vi "Rotating and using Text.vi"() -> ()   [LabVIEW 2023]
doc: "This VI demonstrates how to display text in a 3D Picture with the Create Text with Alignment VI."
uses:
  <vilib>/Utility/miscctls.llb/LVSceneTextAlignment.ctl
  <vilib>/picture/3D Picture Control/Object/Create Object (drawable).vi
  <vilib>/picture/3D Picture Control/Helpers/Apply Texture (no reference).vi
  <vilib>/picture/3D Picture Control/Object/Add Object (no reference).vi
  <vilib>/picture/3D Picture Control/Object/Add Object (reference).vi
  <vilib>/picture/3D Picture Control/NI_3D Picture Control.lvlib
panel:
  in  "Text":string="LabVIEW"
  in  "Stop":bool
  out "3D Picture":refnum<vi>(3d-picture)
  # "Overview: This VI demonstrates how to display text in a 3D Picture with the Create Text with Alignment VI. \nRequirements: LabVIEW Full Development System\nInstructions:\n1. Run the VI. You will see the Text value as a texture on the cube and as several separate objects around the cube.\n2. Click Stop to stop the VI."
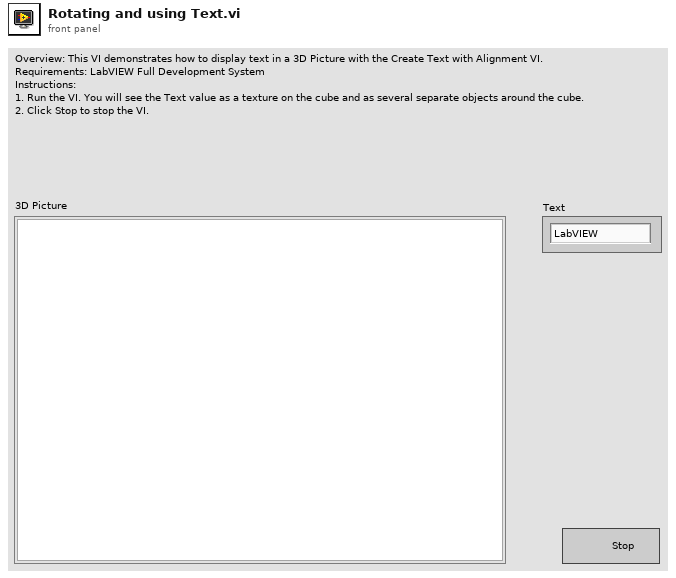
[diagram p1: front panel]
types:
  T1 = typedef "LVSceneTextAlignment.ctl" = cluster{"Horizontal Alignment":enum8{"Left", "Right", "Center"}, "Vertical Alignment":enum8{"Top", "Bottom", "Center", "Base Line", "Bottom Base Line"}}
  T2 = cluster{"Alignment":T1, "Axis Alignment":enum8{"X-Y", "Y-Z", "X-Z", "Reversed X-Y", "Reversed Y-Z", "Reversed X-Z", "Screen"}, "Vertical?":bool, "Wrap Distance":sgl}
  T3 = cluster{"horizontal":enum16{"left", "center", "right"}, "vertical":enum16{"top", "center", "bottom"}}
  T4 = enum16{"As a Decal", "With Modulation", "With Blending", "As a replacement"}
  T5 = cluster{"left":i16, "top":i16, "right":i16, "bottom":i16}
  T6 = typedef "imagedata.ctl" = cluster{"image type":i32, "image depth":i32, "image":u8[], "mask":u8[], "colors":u32[], "Rectangle":cluster{"left":i16, "top":i16, "right":i16, "bottom":i16}}
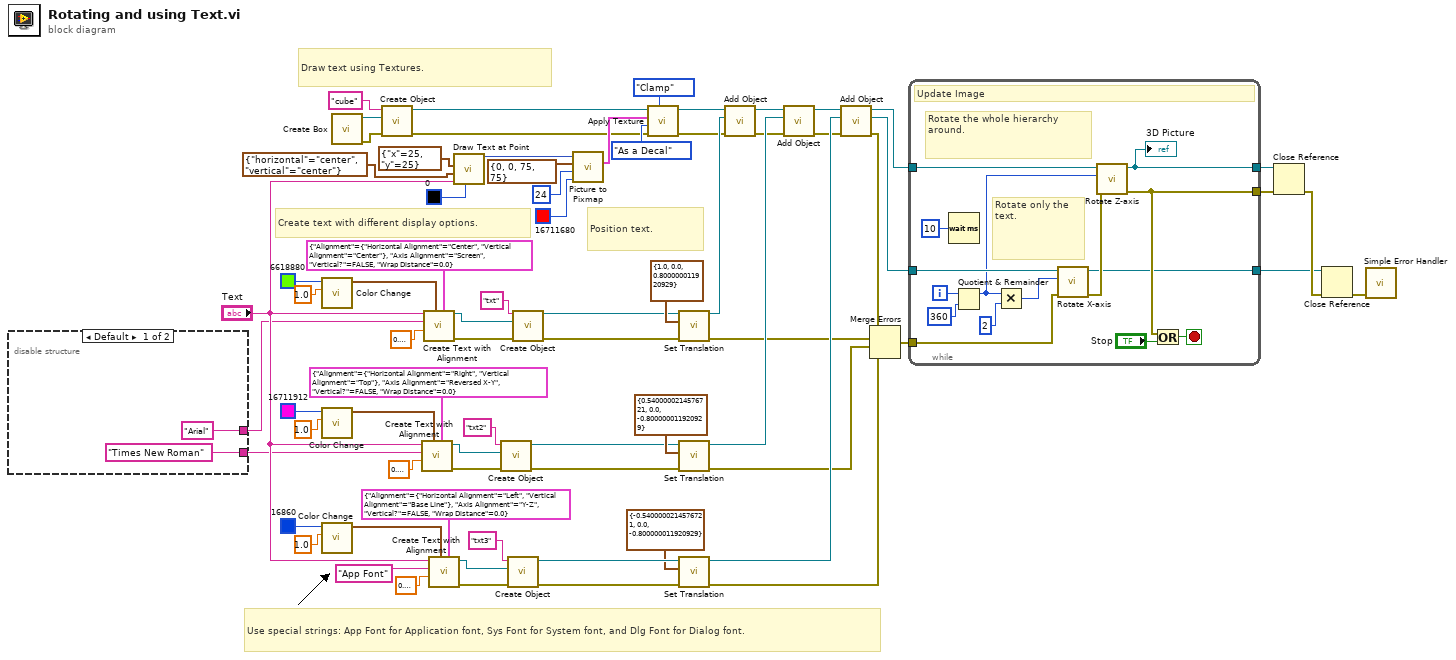
[diagram p0: block diagram]
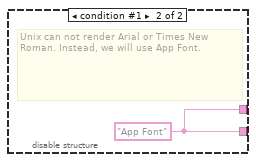
[diagram p2: hidden frame]
diagram:
  # "Use special strings: App Font for Application font, Sys Font for System font, and Dlg Font for Dialog font."
  # "Create text with different display options."
  # "Position text."
  # "Draw text using Textures."
  n1 = disable-structure shown="Default" {
    disable-tunnel: ["Arial" ("pattern") w76] -> w2
    disable-tunnel: ["Times New Roman" ("pattern") w76] -> w1
    frame condition #0 (active) {
    }
    frame condition #1 {
      w76 = "App Font" ("pattern")
      # "Unix can not render Arial or Times New Roman. Instead, we will use App Font."
    }
  }
  n2 = call <vilib>:"Color Change.vi"("Alpha"=1.0, "Color"=u32 6618880) -> ("RGBA"=w70:cluster{"R":sgl, "G":sgl, "B":sgl, "A":sgl})  [unwired: 9 in]
  n3 = call <vilib>:"Color Change.vi"("Alpha"=1.0, "Color"=u32 16711912) -> ("RGBA"=w46:cluster{"R":sgl, "G":sgl, "B":sgl, "A":sgl})  [unwired: 9 in]
  n4 = call <vilib>:"Color Change.vi"("Alpha"=1.0, "Color"=u32 16860) -> ("RGBA"=w33:cluster{"R":sgl, "G":sgl, "B":sgl, "A":sgl})  [unwired: 9 in]
  n5 = call <vilib>:"Create Box.vi"() -> ("error out"=w24:errorcluster, "New Box Refnum"=w73:refnum<vi>)  [unwired: 10 in]
  n6 = call-poly <vilib>:"Create Object.vi"("error in (no error)"=w24, "Geometry"=w73, "Name"="cube") -> ("error out"=w23:errorcluster, "Scene:New Object"=w57:refnum<vi>)  [unwired: 7 in]
  n7 = call <vilib>:"Create Text with Alignment.vi"("Font Options"=T2 {"Alignment"={"Horizontal Alignment"=enum."Right", "Vertical Alignment"=enum."Top"}, "Axis Alignment"=enum."Reversed X-Y", "Vertical?"=FALSE, "Wrap Distance"=0.0} ("Font options"), "Color"=w46, "Character Size"=sgl 0.3, "Font Name"=w1, "Text"="Text") -> ("error out"=w16:errorcluster, "New Text Refnum"=w42:refnum<vi>)  [unwired: 5 in]
  n8 = call <vilib>:"Create Text with Alignment.vi"("Font Options"=T2 {"Alignment"={"Horizontal Alignment"=enum."Center", "Vertical Alignment"=enum."Center"}, "Axis Alignment"=enum."Screen", "Vertical?"=FALSE, "Wrap Distance"=0.0} ("Font options"), "Color"=w70, "Character Size"=sgl 0.2, "Font Name"=w2, "Text"="Text") -> ("error out"=w18:errorcluster, "New Text Refnum"=w55:refnum<vi>)  [unwired: 5 in]
  n9 = call <vilib>:"Create Text with Alignment.vi"("Font Options"=T2 {"Alignment"={"Horizontal Alignment"=enum."Left", "Vertical Alignment"=enum."Base Line"}, "Axis Alignment"=enum."Y-Z", "Vertical?"=FALSE, "Wrap Distance"=0.0} ("Font options"), "Color"=w33, "Character Size"=sgl 0.2, "Font Name"="App Font" ("pattern"), "Text"="Text") -> ("error out"=w14:errorcluster, "New Text Refnum"=w36:refnum<vi>)  [unwired: 5 in]
  n10 = call <vilib>:"Draw Text at Point.vi"("text color(black)"=u32 0, "text"="Text", "alignment(left, top)"=T3 {"horizontal"=enum."center", "vertical"=enum."center"}, "origin"=cluster{"x":i16, "y":i16} {"x"=25, "y"=25}) -> ("new picture"=w63:picture)  [unwired: 6 in, 1 out]
  n11 = call-poly <vilib>:"Create Object.vi"("error in (no error)"=w16, "Geometry"=w42, "Name"="txt2") -> ("error out"=w15:errorcluster, "Scene:New Object"=w41:refnum<vi>)  [unwired: 7 in]
  n12 = call-poly <vilib>:"Create Object.vi"("error in (no error)"=w14, "Geometry"=w36, "Name"="txt3") -> ("error out"=w13:errorcluster, "Scene:New Object"=w37:refnum<vi>)  [unwired: 7 in]
  n13 = call-poly <vilib>:"Create Object.vi"("error in (no error)"=w18, "Geometry"=w55, "Name"="txt") -> ("error out"=w17:errorcluster, "Scene:New Object"=w54:refnum<vi>)  [unwired: 7 in]
  n14 = call <vilib>:"Picture to Pixmap.vi"("Background Color"=u32 16711680, "depth"=24, "rect"=T5 {"left"=0, "top"=0, "right"=75, "bottom"=75}, "picture"=w63) -> ("image data"=w64:T6)  [unwired: 6 in, 1 out]
  n15 = call-poly <vilib>:"Apply Texture.vi"("Horizontal Wrap Mode"=enum16{"Clamp", "Repeat"}."Clamp", "error in (no error)"=w23, "Apply Mode"=T4."As a Decal", "Image Data"=w64, "Scene Object In"=w57) -> ("error out"=w22:errorcluster, "Scene Object Out"=w56:refnum<vi>)  [unwired: 5 in]
  n16 = call <vilib>:"Set Translation.vi"("error in (no error)"=w17, "Translation"=cluster{"X":sgl, "Y":sgl, "Z":sgl} {"X"=1.0, "Y"=0.0, "Z"=0.8}, "Scene Object"=w54) -> ("error out"=w12:errorcluster, "Translated Object"=w66:refnum<vi>)  [unwired: 7 in]
  n17 = call <vilib>:"Set Translation.vi"("error in (no error)"=w15, "Translation"=cluster{"X":sgl, "Y":sgl, "Z":sgl} {"X"=0.54, "Y"=0.0, "Z"=-0.8}, "Scene Object"=w41) -> ("error out"=w11:errorcluster, "Translated Object"=w40:refnum<vi>)  [unwired: 7 in]
  n18 = call <vilib>:"Set Translation.vi"("error in (no error)"=w13, "Translation"=cluster{"X":sgl, "Y":sgl, "Z":sgl} {"X"=-0.54, "Y"=0.0, "Z"=-0.8}, "Scene Object"=w37) -> ("error out"=w10:errorcluster, "Translated Object"=w25:refnum<vi>)  [unwired: 7 in]
  n19 = call-poly <vilib>:"Add Object.vi"("error in (no error)"=w22, "New Object In"=w66, "Scene Object In"=w56) -> ("error out"=w21:errorcluster, "Scene Object Out"=w45:refnum<vi>)  [unwired: 7 in]
  n20 = call-poly <vilib>:"Add Object.vi"("error in (no error)"=w21, "New Object In"=w40, "Scene Object In"=w45) -> ("error out"=w20:errorcluster, "Scene Object Out"=w27:refnum<vi>)  [unwired: 7 in]
  n21 = call-poly <vilib>:"Add Object.vi"("error in (no error)"=w20, "New Object In"=w25, "Scene Object In"=w27) -> ("error out"=w9:errorcluster, "New Object Out"=w19:refnum<vi>, "Scene Object Out"=w26:refnum<vi>)  [unwired: 6 in]
  n22 = Merge Errors(w9, w12, w11, w10) -> (w8:errorcluster)
  n23 = while {
    tunnel: w26 -> [w87]
    tunnel: w19 -> [w86]
    tunnel: w8 -> [w82]
    tunnel: [w79] -> w7
    tunnel: [w78] -> w4
    tunnel: [w77] -> w3
    i -> [w88]
    stop <- w80 stop-if-true
    # "Rotate only the text."
    # "Rotate the whole hierarchy around."
    # "Update Image"
    n24 = Wait (ms)(milliseconds to wait=u32 10 ("millisecond multiple")) -> ()  [unwired: 1 out]
    n25 = Quotient & Remainder(x=w88, y=360) -> (x-y*floor(x/y)=w85:i32)  [unwired: 1 out]
    n26 = Multiply(x=w85, y=2) -> (x*y=w84:i32)
    n27 = call <vilib>:"Rotate X-axis.vi"("error in (no error)"=w82, "angle"=w84, "Scene Object In"=w86) -> ("error out"=w81:errorcluster, "Scene Object Out"=w78:refnum<vi>)  [unwired: 7 in]
    n28 = call <vilib>:"Rotate Z-axis.vi"("error in (no error)"=w81, "angle"=w85, "Scene Object In"=w87) -> ("error out"=w79:errorcluster, "Scene Object Out"=w77:refnum<vi>)  [unwired: 7 in]
    "3D Picture" <- w77
    n29 = Or(x=w79, y="Stop") -> (x .or. y?=w80:bool)
  }
  n30 = Close Reference(reference=w3, error in (no error)=w7) -> (error out=w5:errorcluster)
  n31 = Close Reference(reference=w4, error in (no error)=w5) -> (error out=w6:errorcluster)
  n32 = call <vilib>:"Simple Error Handler.vi"("error in (no error)"=w6) -> ()  [unwired: 4 in, 5 out]
